vi "Async.vi"(7 "command":T1, 8 "error in (no error)":errorcluster, 9 "framework iteration":u64, 10 "Dispatcher Interface in":refnum<class "Dispatcher Interface.lvclass">, 11 "Plugin Timing Bundle in":refnum<class "Scheduler Plugin Bundle.lvclass">) -> (0 "error out":errorcluster, 2 "Dispatcher Interface out":refnum<class "Dispatcher Interface.lvclass">, 3 "Plugin Timing Bundle out":refnum<class "Scheduler Plugin Bundle.lvclass">)   [LabVIEW 2017, in "Scheduler Plugin Bundle.lvclass"]
uses:
  Scheduler/Scheduler Plugin Bundle.lvclass
  Timing.lvclass
  Scheduler/Scheduler Transfer Group Bundle.lvclass
  Interfaces/Dispatcher/Dispatcher Interface.lvclass
  Interfaces/Dispatcher/Command.ctl
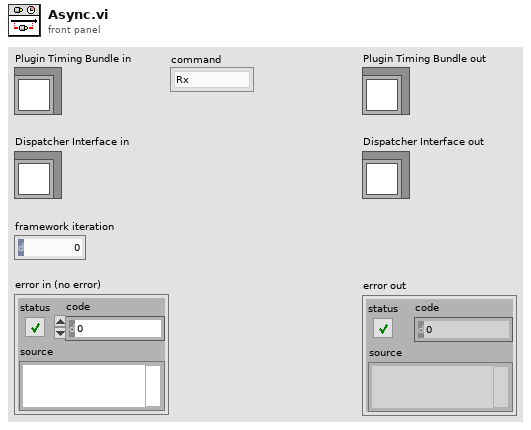
[diagram p1: front panel]
types:
  T1 = typedef "DSF Core.lvlib/Dispatcher Interface.lvclass/Command.ctl" = enum8{"Rx", "Tx", "Set Inline Buffer", "Shutdown"}
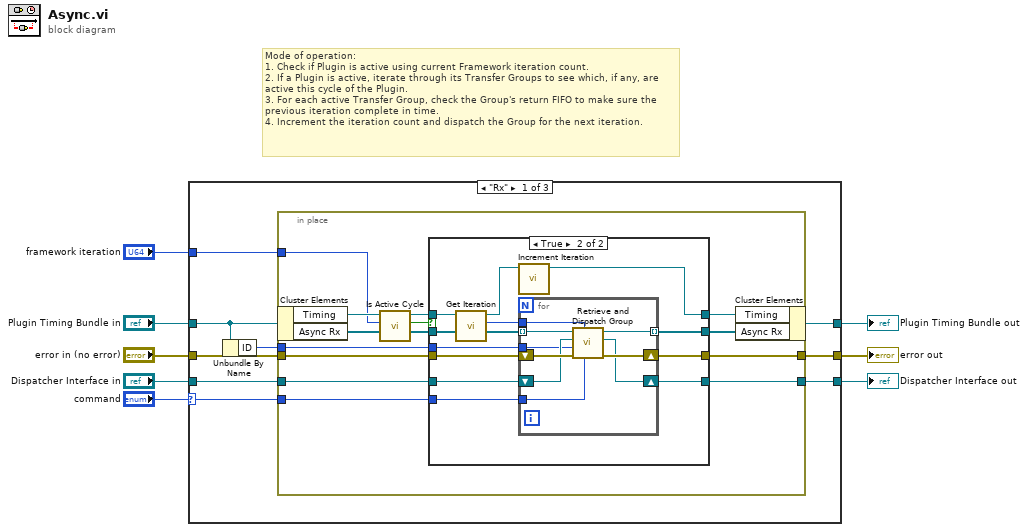
[diagram p0: block diagram]
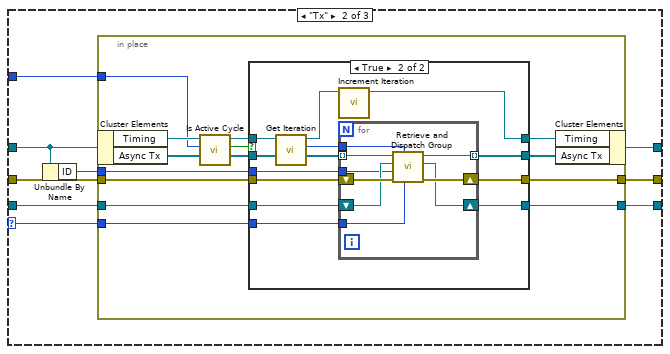
[diagram p3: hidden frame]
diagram:
  # "Mode of operation:\n1. Check if Plugin is active using current Framework iteration count.\n2. If a Plugin is active, iterate through its Transfer Groups to see which, if any, are active this cycle of the Plugin.\n3. For each active Transfer Group, check the Group's return FIFO to make sure the previous iteration complete in time.\n4. Increment the iteration count and dispatch the Group for the next iteration."
  n1 = case shown="\"Rx\"" "command" {
    selector: "command" -> [w9 w56 _]
    tunnel: "Dispatcher Interface in" -> [w17 w64 w103]
    tunnel: [w16 w63 w103] -> w7
    tunnel: "error in (no error)" -> [w15 w62 w104]
    tunnel: [w14 w61 w104] -> w5
    tunnel: "framework iteration" -> [w13 w60 _]
    tunnel: [w12 w59 w105] -> w3
    tunnel: "Plugin Timing Bundle in" -> [w11 w58 w105]
    frame "Rx" {
      n2 = Unbundle By Name(w11) -> ("ID"=w10:i32)
      n3 = in-place {
        in-place-border: w17 -> [w30]
        in-place-border: [w29] -> w16
        in-place-border: w15 -> [w28]
        in-place-border: [w27] -> w14
        in-place-border: w13 -> [w20]
        in-place-border: w10 -> [w21]
        in-place-border: w9 -> [w18]
        n4 = in-place-cluster #1(w11) -> ("Timing"=w23:refnum<class "Timing.lvclass">, "Async Rx"=w24:refnum<class "Scheduler Transfer Group Bundle.lvclass">[])
        n5 = call "Is Active Cycle.vi"("iteration"=w20, "Timing in"=w23) -> ("active?"=w26:bool, "Timing out"=w25:refnum<class "Timing.lvclass">)  [unwired: 8 in]
        n6 = case shown="True" w26 {
          tunnel: [w32 w38] -> w22
          tunnel: w30 -> [w34 w46]
          tunnel: [w34 w45] -> w29
          tunnel: w28 -> [w33 w44]
          tunnel: [w33 w43] -> w27
          tunnel: w21 -> [_ w42]
          tunnel: w24 -> [w32 w41]
          tunnel: w25 -> [w31 w37]
          tunnel: [w31 w36] -> w19
          tunnel: w18 -> [_ w35]
          frame False {
          }
          frame True {
            n7 = call "Get Iteration.vi"("Timing in"=w37) -> ("Iteration"=w40:u64, "Timing out"=w39:refnum<class "Timing.lvclass">)  [unwired: 9 in]
            n8 = call "Increment Iteration.vi"("Timing in"=w39) -> ("Timing out"=w36:refnum<class "Timing.lvclass">)  [unwired: 10 in]
            n9 = for {
              tunnel: w41 -> [w55] mode=indexing
              tunnel: [w52] -> w38 mode=indexing
              shift-right: [w50] -> w45
              shift-left: w46 -> [w51]
              shift-right: [w53] -> w43
              shift-left: w44 -> [w54]
              tunnel: w42 -> [w49]
              tunnel: w40 -> [w48]
              tunnel: w35 -> [w47]
              n10 = call "Retrieve and Dispatch Group.vi"("command"=w47, "plugin iteration"=w48, "error in (no error)"=w54, "plugin ID"=w49, "Dispatcher Interface in"=w51, "Scheduler Transfer Group Bundle in"=w55) -> ("error out"=w53:errorcluster, "Dispatcher Interface out"=w50:refnum<class "Dispatcher Interface.lvclass">, "Scheduler Transfer Group Bundle out"=w52:refnum<class "Scheduler Transfer Group Bundle.lvclass">)  [unwired: 3 in]
            }
          }
        }
        n11 = in-place-cluster #1("Timing"=w19, "Async Rx"=w22) -> (w12:refnum<class "Scheduler Plugin Bundle.lvclass">)
      }
    }
    frame "Tx" {
      n12 = Unbundle By Name(w58) -> ("ID"=w57:i32)
      n13 = in-place {
        in-place-border: w64 -> [w77]
        in-place-border: [w76] -> w63
        in-place-border: w62 -> [w75]
        in-place-border: [w74] -> w61
        in-place-border: w60 -> [w67]
        in-place-border: w57 -> [w68]
        in-place-border: w56 -> [w65]
        n14 = in-place-cluster #2(w58) -> ("Timing"=w70:refnum<class "Timing.lvclass">, "Async Tx"=w71:refnum<class "Scheduler Transfer Group Bundle.lvclass">[])
        n15 = call "Is Active Cycle.vi"("iteration"=w67, "Timing in"=w70) -> ("active?"=w73:bool, "Timing out"=w72:refnum<class "Timing.lvclass">)  [unwired: 8 in]
        n16 = case shown="True" w73 {
          tunnel: [w79 w85] -> w69
          tunnel: w77 -> [w81 w93]
          tunnel: [w81 w92] -> w76
          tunnel: w75 -> [w80 w91]
          tunnel: [w80 w90] -> w74
          tunnel: w68 -> [_ w89]
          tunnel: w71 -> [w79 w88]
          tunnel: w72 -> [w78 w84]
          tunnel: [w78 w83] -> w66
          tunnel: w65 -> [_ w82]
          frame False {
          }
          frame True {
            n17 = call "Get Iteration.vi"("Timing in"=w84) -> ("Iteration"=w87:u64, "Timing out"=w86:refnum<class "Timing.lvclass">)  [unwired: 9 in]
            n18 = call "Increment Iteration.vi"("Timing in"=w86) -> ("Timing out"=w83:refnum<class "Timing.lvclass">)  [unwired: 10 in]
            n19 = for {
              tunnel: w88 -> [w102] mode=indexing
              tunnel: [w99] -> w85 mode=indexing
              shift-right: [w97] -> w92
              shift-left: w93 -> [w98]
              shift-right: [w100] -> w90
              shift-left: w91 -> [w101]
              tunnel: w89 -> [w96]
              tunnel: w87 -> [w95]
              tunnel: w82 -> [w94]
              n20 = call "Retrieve and Dispatch Group.vi"("command"=w94, "plugin iteration"=w95, "error in (no error)"=w101, "plugin ID"=w96, "Dispatcher Interface in"=w98, "Scheduler Transfer Group Bundle in"=w102) -> ("error out"=w100:errorcluster, "Dispatcher Interface out"=w97:refnum<class "Dispatcher Interface.lvclass">, "Scheduler Transfer Group Bundle out"=w99:refnum<class "Scheduler Transfer Group Bundle.lvclass">)  [unwired: 3 in]
            }
          }
        }
        n21 = in-place-cluster #2("Timing"=w66, "Async Tx"=w69) -> (w59:refnum<class "Scheduler Plugin Bundle.lvclass">)
      }
    }
    frame "Shutdown", Default {
    }
  }
  "Plugin Timing Bundle out" <- w3
  "Dispatcher Interface out" <- w7
  "error out" <- w5
